vi "oax_Set Transition Pattern (block).vi"(5 "acc transition ratio":dbl=0.05, 7 "reset?":bool=TRUE, 9 "block size":dbl, 10 "time period":dbl[](array[numeric]), 11 "speed":dbl[](array[numeric])) -> (3 "current speed positions":T1(array[cluster]))   [LabVIEW 2017]
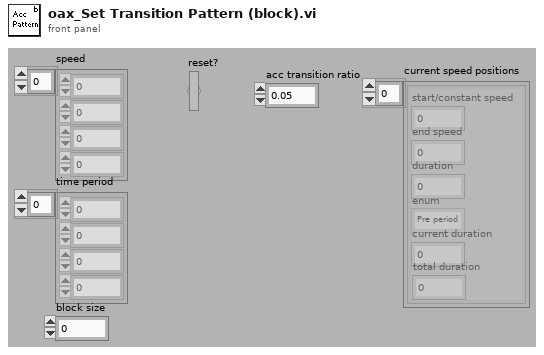
[diagram p1: front panel]
types:
  T1 = cluster{"start/constant speed":dbl, "end speed":dbl, "duration":dbl, "enum":enum16{"Pre period", "Middle period", "Post period"}, "current duration":dbl, "total duration":dbl}[]
  T2 = cluster{"start speed":dbl, "end speed":dbl, "duration":dbl, "start time":dbl, "mode":enum16{"Pre period", "Middle period", "Post period"}, "total duration":dbl}[]
  T3 = cluster{"start speed":dbl, "end speed":dbl, "duration":dbl, "start time":dbl, "mode":enum16{"Pre period", "Middle period", "Post period"}, "total duration":dbl}
  T4 = enum16{"Pre period", "Middle period", "Post period"}
  T5 = cluster{"start speed":dbl, "end speed":dbl, "duration":dbl, "mode":enum16{"Pre period", "Middle period", "Post period"}, "block size":dbl, "total duration":dbl}
  T6 = cluster{"start speed":dbl, "end speed":dbl, "duration":dbl, "mode":enum16{"Pre period", "Middle period", "Post period"}, "block size":dbl, "total duration":dbl}[]
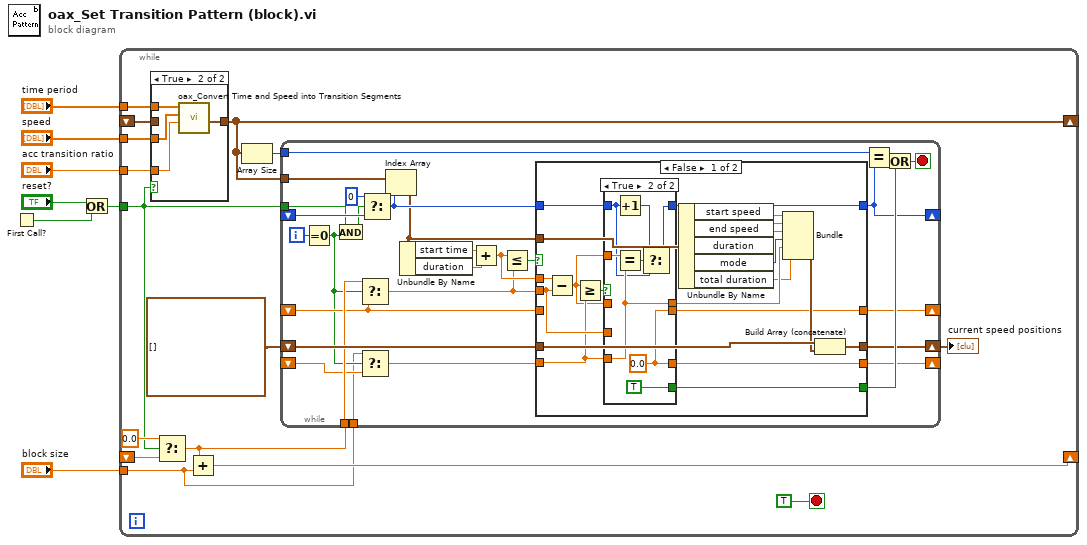
[diagram p0: block diagram]
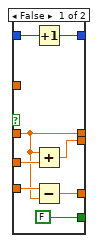
[diagram p2: hidden frame]
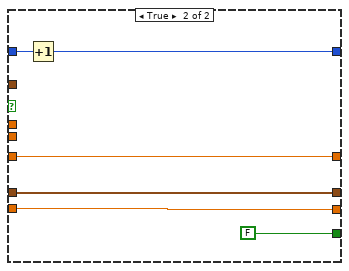
[diagram p3: hidden frame]
diagram:
  n1 = First Call?() -> (First Call?: T/F=w4:bool)
  n2 = Or(x="reset?", y=w4) -> (x .or. y?=w3:bool)
  n3 = while {
    tunnel: "time period" -> [w22]
    tunnel: "speed" -> [w21]
    tunnel: w3 -> [w14]
    shift-right: [w13] -> _
    shift-left: _ -> [w18]
    tunnel: "block size" -> [w8]
    tunnel: "acc transition ratio" -> [w16]
    shift-right: [w12] -> _
    shift-left: _ -> [w17]
    stop <- TRUE stop-if-true
    n4 = case shown="True" w14 {
      tunnel: w22 -> [_ w96]
      tunnel: w21 -> [_ w97]
      tunnel: [w93 w94] -> w12
      tunnel: w17 -> [w93 _]
      tunnel: w16 -> [_ w95]
      frame False {
      }
      frame True {
        n5 = call <vilib>:"oax_Convert Time and Speed into Transition Segments.vi"("acc transition ratio"=w95, "speed"=w97, "time period"=w96) -> ("data in speed segments"=w94:T2)  [unwired: 8 in]
      }
    }
    n6 = Select(t=0.0, s=w14, f=w18) -> (s? t:f=w15:dbl)
    n7 = Add(x=w15, y=w8) -> (x+y=w13:dbl)
    n8 = Array Size(array=w12) -> (size(s)=w11:i32)
    n9 = while {
      tunnel: w12 -> [w50]
      shift-right: [w40] -> _
      shift-left: _ -> [w49]
      tunnel: w15 -> [w29]
      tunnel: w14 -> [w33]
      tunnel: w11 -> [w45]
      shift-right: [w38] -> w9
      shift-left: T1 [] ("current speed positions") -> [w39]
      tunnel: w8 -> [w23]
      shift-right: [w31] -> _
      shift-left: _ -> [w28]
      shift-right: [w27] -> _
      shift-left: _ -> [w25]
      i -> [w34]
      stop <- w42 stop-if-true
      n10 = Equal To 0?(x=w34) -> (x = 0?=w26:bool)
      n11 = And(x=w33, y=w26) -> (x .and. y?=w32:bool)
      n12 = Select(t=w29, s=w26, f=w28) -> (s? t:f=w30:dbl)
      n13 = Select(t=w23, s=w26, f=w25) -> (s? t:f=w24:dbl)
      n14 = Select(t=0, s=w32, f=w49) -> (s? t:f=w41:i32)
      n15 = Index Array(array=w50, index=w41) -> (element=w37:T3)
      n16 = Unbundle By Name(w37) -> ("start time"=w47:dbl, "duration"=w36:dbl)
      n17 = Add(x=w47, y=w36) -> (x+y=w35:dbl)
      n18 = Less Or Equal?(x=w35, y=w30) -> (x <= y?=w46:bool)
      n19 = case shown="False" w46 {
        tunnel: [w59 FALSE] -> w43
        tunnel: w41 -> [w61 w91]
        tunnel: [w60 w90] -> w40
        tunnel: w39 -> [w68 w89]
        tunnel: [w67 w89] -> w38
        tunnel: w37 -> [w70 _]
        tunnel: w35 -> [w56 _]
        tunnel: w30 -> [w55 _]
        tunnel: [w57 w88] -> w31
        tunnel: w28 -> [_ w88]
        tunnel: [w54 w87] -> w27
        tunnel: w24 -> [w53 w87]
        frame False {
          n20 = Subtract(x=w56, y=w55) -> (x-y=w52:dbl)
          n21 = Greater Or Equal?(x=w52, y=w53) -> (x >= y?=w62:bool)
          n22 = case shown="True" w62 {
            tunnel: w61 -> [w78 w80]
            tunnel: [w76 w79] -> w60
            tunnel: [FALSE TRUE] -> w59
            tunnel: w53 -> [w73 w83]
            tunnel: [w72 w83] -> w58
            tunnel: w52 -> [w72 _]
            tunnel: [w74 w85] -> w57
            tunnel: w55 -> [w75 _]
            tunnel: [w71 w85] -> w54
            tunnel: w52 -> [_ w84]
            frame False {
              n23 = Increment(x=w78) -> (x+1=w76:i32)
              n24 = Add(x=w72, y=w75) -> (x+y=w74:dbl)
              n25 = Subtract(x=w73, y=w72) -> (x-y=w71:dbl)
            }
            frame True {
              w85 = 0.0
              n26 = Increment(x=w80) -> (x+1=w81:i32)
              n27 = Equal?(x=w84, y=w83) -> (x = y?=w82:bool)
              n28 = Select(t=w81, s=w82, f=w80) -> (s? t:f=w79:i32)
            }
          }
          n29 = Unbundle By Name(w70) -> ("start speed"=w69:dbl, "end speed"=w63:dbl, "duration"=w64:dbl, "mode"=w65:T4, "total duration"=w51:dbl)
          n30 = Bundle("start speed"=w69, "end speed"=w63, "duration"=w64, "mode"=w65, "block size"=w58, "total duration"=w51) -> (w66:T5)  [unwired: 1 in]
          n31 = Build Array (concatenate)(w68, w66) -> (w67:T6)
        }
        frame True {
          n32 = Increment(x=w91) -> (x+1=w90:i32)
        }
      }
      n33 = Equal?(x=w45, y=w40) -> (x = y?=w44:bool)
      n34 = Or(x=w44, y=w43) -> (x .or. y?=w42:bool)
    }
    "current speed positions" <- w9
  }
